vi "GetValue.vi"(5 "cmd":string, 6 "error in":errorcluster, 9 "connection ID":refnum<k5>) -> (0 "error out":errorcluster, 3 "connection ID out":refnum<k5>, 4 "value":string)   [LabVIEW 2014, in "Raspberry Pi Compatible Compiler for LabVIEW.lvlib" / "RasPiDownloader.lvlib"]
uses:
  RasPiDownloader.lvlib
  Websocket/Websocket.lvlib
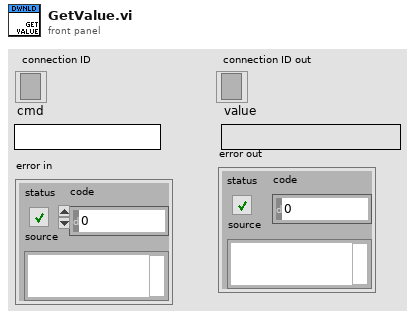
[diagram p1: front panel]
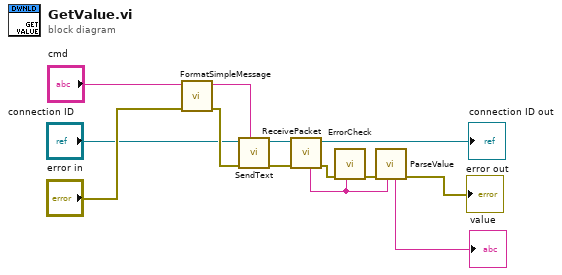
[diagram p0: block diagram]
diagram:
  n1 = call "FormatSimpleMessage.vi"("error in"="error in", "cmd"="cmd") -> ("error out"=w9:errorcluster, "JSON string"=w10:string)  [unwired: 8 in]
  n2 = call "SendText.vi"("payload"=w10, "error in"=w9, "connection ID"="connection ID") -> ("error out"=w11:errorcluster, "connection ID out"=w12:refnum<k5>)  [unwired: 5 in]
  n3 = call "ReceivePacket.vi"("error in"=w11, "connection ID"=w12) -> ("error out"=w13:errorcluster, "connection ID out"=→"connection ID out":refnum<k5>, "payload"=w6:string)  [unwired: 5 in]
  n4 = call "ErrorCheck.vi"("payload"=w6, "error in"=w13) -> ("error out"=w7:errorcluster)  [unwired: 7 in]
  n5 = call "ParseValue.vi"("payload"=w6, "error in"=w7) -> ("error out"=→"error out":errorcluster, "value"=→"value":string)  [unwired: 6 in]
